vi "Periodic Tasks.vi"(8 "error in":errorcluster) -> ()   [LabVIEW 2013]
doc: "This VI runs in parallel to other tasks. It can contain as many user-defined periodic loops as you need. These can carry out PID or other sorts of timed response."
uses:
  <vilib>/Rock Robotics/SystemInterfaces/Utilities/FPGA_UtilitiesLED Source.ctl
  <vilib>/Rock Robotics/SystemInterfaces/Utilities/FPGA_UtilitiesLED State.ctl
  <vilib>/Rock Robotics/WPI/DriverStation/DriverStationLCD/WPI_DriverStationLCDLCDLine.ctl
  Robot Global Data.vi
panel:
  in  "DesiredPos 2":dbl
  in  "Deadband 2":dbl=0.2
  in  "P Gain 2":dbl=1.0
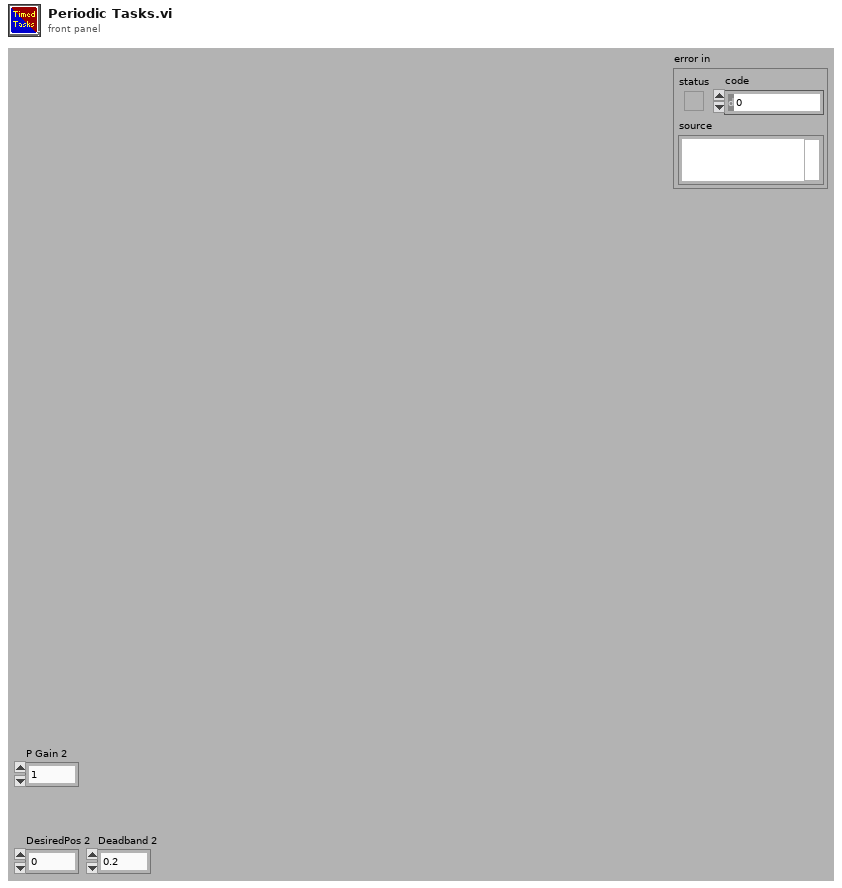
[diagram p1: front panel]
types:
  T1 = typedef "WPI_AnalogChannelDevRef.ctl" = cluster{"DevStatus":errorcluster, "Analog Module":T2, "Analog Channel":T3}
  T2 = typedef "FPGA_TypedefAnalogModule.ctl" = enum16{"Analog Module 1", "Analog Module 2"}
  T3 = typedef "FPGA_AIChannel.ctl" = enum8{"AI 1", "AI 2", "AI 3", "AI 4", "AI 5", "AI 6", "AI 7", "AI 8", "Invalid"}
  T4 = typedef "WPI_DigitalInputDevRef.ctl" = cluster{"DevStatus":errorcluster, "DIO Channel":T5, "Digital Module":T6}
  T5 = typedef "FPGA_DIOChannel.ctl" = enum8{"DIO 1", "DIO 2", "DIO 3", "DIO 4", "DIO 5", "DIO 6", "DIO 7", "DIO 8", "DIO 9", "DIO 10", "DIO 11", "DIO 12", "DIO 13", "DIO 14", "Invalid"}
  T6 = typedef "FPGA_TypedefDigitalModule.ctl" = enum16{"Digital Module 1", "Digital Module 2"}
  T7 = typedef "WPI_EncoderDevRef.ctl" = cluster{"DevStatus":errorcluster, "EncoderIndex":T8, "CounterIndex":T9, "DistancePerCount":dbl, "Decoding Type":T10}
  T8 = typedef "FPGA_EncoderIdx.ctl" = enum8{"Enc 0", "Enc 1", "Enc 2", "Enc 3", "Invalid"}
  T9 = typedef "FPGA_CounterCtrSystemIndex.ctl" = enum8{"Ctr 0", "Ctr 1", "Ctr 2", "Ctr 3", "Ctr 4", "Ctr 5", "Ctr 6", "Ctr 7", "Invalid"}
  T10 = typedef "WPI_EncoderType.ctl" = enum16{"1x", "2x", "4x"}
  T11 = cluster{"Winch Desired Location":dbl, "Winch Desired Location 2":dbl, "Winch Desired Location 3":dbl}
  T12 = typedef "FPGA_UtilitiesLED State.ctl" = enum16{"Off", "On", "Toggle"}
  T13 = typedef "FPGA_UtilitiesLED Source.ctl" = enum16{"User LED", "FPGA LED"}
  T14 = typedef "WPI_DriverStationLCDLCDLine.ctl" = enum16{"Main - Line 1", "User - Line 2", "User - Line 3", "User - Line 4", "User - Line 5", "User - Line 6"}
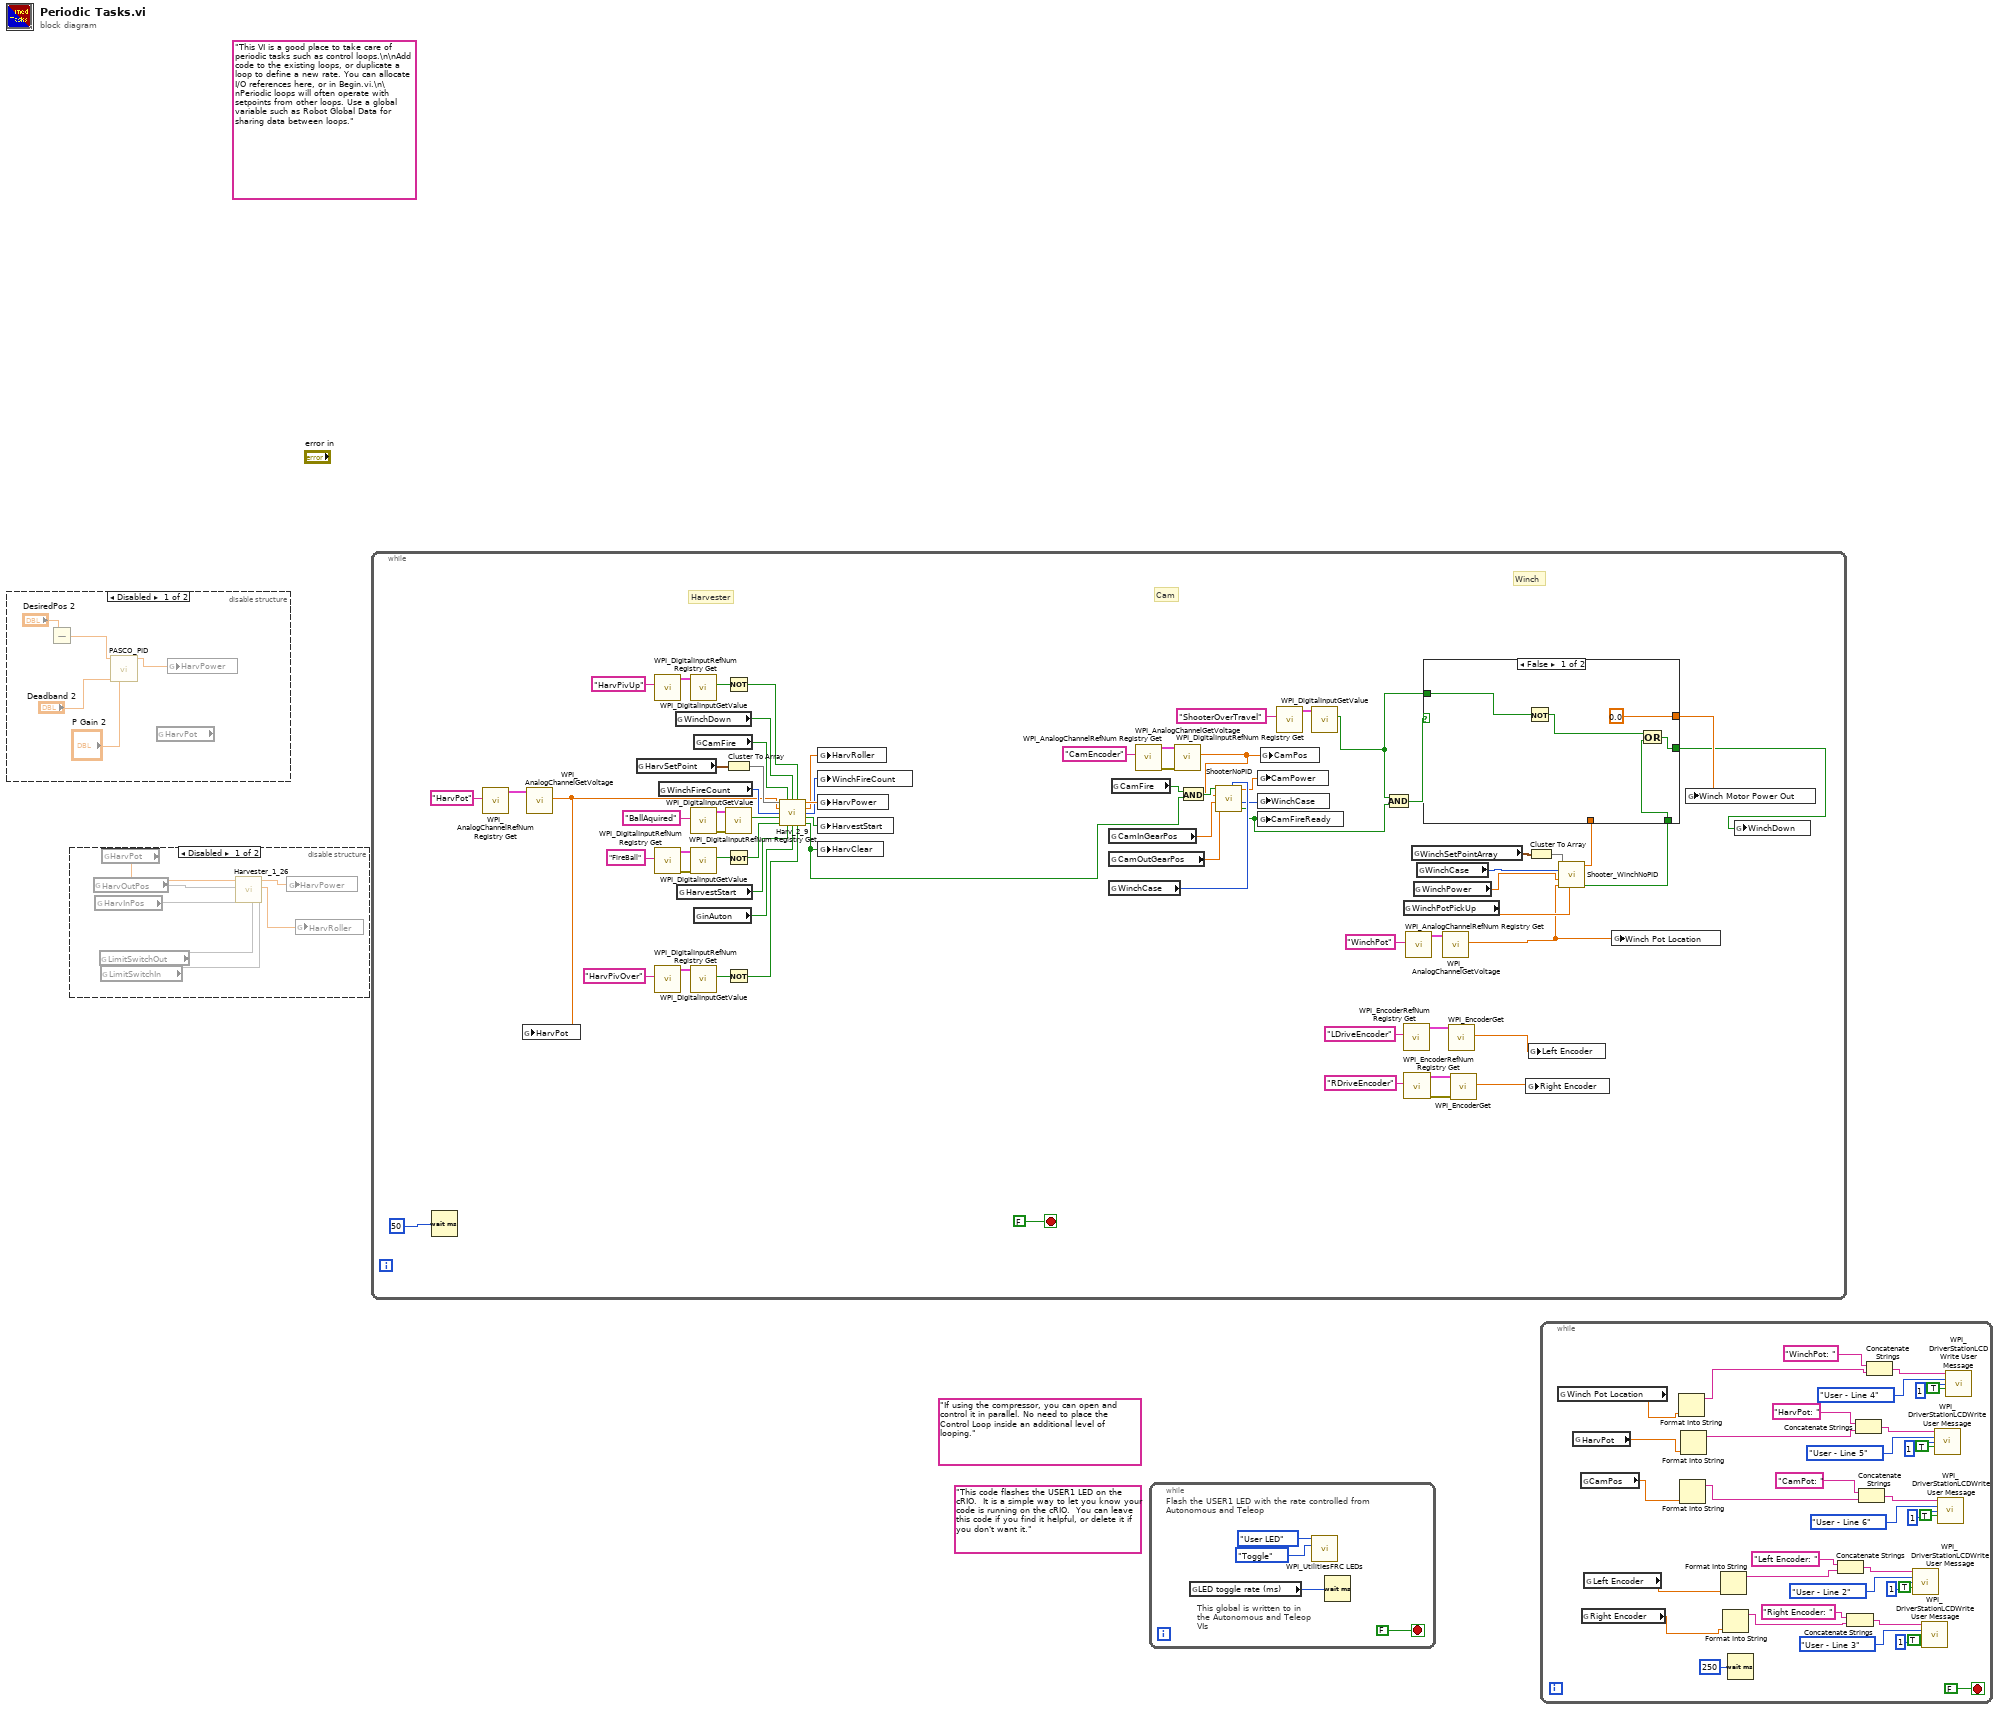
[diagram p0: block diagram]
diagram:
  (unwired) "If using the compressor, you can open and control it in parallel. No need to place the Control Loop inside an additional level of looping."
  (unwired) "This code flashes the USER1 LED on the cRIO.  It is a simple way to let you know your code is running on the cRIO.  You can leave this code if you find it helpful, or delete it if you don't want it."
  (unwired) "This VI is a good place to take care of periodic tasks such as control loops.\n\nAdd code to the existing loops, or duplicate a loop to define a new rate. You can allocate I/O references here, or in Begin.vi.\n\nPeriodic loops will often operate with setpoints from other loops. Use a global variable such as Robot Global Data for sharing data between loops."
  n1 = disable-structure shown="Disabled" {
    frame Disabled {
      n2 = Subtract(x="DesiredPos 2") -> (y=w6:dbl, x-y=w1:dbl)
      n3 = call "PASCO_PID.vi"("Delta"=w1, "Deadband"="Deadband 2", "P Gain"="P Gain 2") -> ("Output"=w3:dbl)  [unwired: 11 in, 1 out]
      n4 = global read "Robot Global Data.vi" "HarvPot"() -> (w5:dbl)
      n5 = global write "Robot Global Data.vi" "HarvPower"(w3) -> ()
    }
    frame Enabled {
    }
  }
  n6 = disable-structure shown="Disabled" {
    frame Disabled {
      n7 = global read "Robot Global Data.vi" "HarvOutPos"() -> (w13)
      n8 = global read "Robot Global Data.vi" "HarvInPos"() -> (w12)
      n9 = global read "Robot Global Data.vi" "LimitSwitchOut"() -> (w11)
      n10 = global read "Robot Global Data.vi" "LimitSwitchIn"() -> (w10)
      n11 = global read "Robot Global Data.vi" "HarvPot"() -> (w14:dbl)
      n12 = call "Harvester_1_26.vi"("LimitSwitchIn"=w10, "LimitSwitchOut"=w11, "HarvInPos"=w12, "HarvOutPos"=w13, "HarvPot"=w14) -> ("HarvRoller"=w9:dbl, "HarvPower"=w8:dbl)  [unwired: 5 in]
      n13 = global write "Robot Global Data.vi" "HarvPower"(w8) -> ()
      n14 = global write "Robot Global Data.vi" "HarvRoller"(w9) -> ()
    }
    frame Enabled {
    }
  }
  n15 = while {
    stop <- FALSE stop-if-true
    # "Winch"
    # "Cam"
    # "Harvester"
    n16 = Wait (ms)(milliseconds to wait=u32 50) -> ()  [unwired: 1 out]
    n17 = call <vilib>:"WPI_AnalogChannelRefNum Registry Get.vi"("refnum name"="HarvPot") -> ("AIDeviceRef"=w82:T1)  [unwired: 9 in, 1 out]
    n18 = call <vilib>:"WPI_AnalogChannelGetVoltage.vi"("AIDeviceRef"=w82) -> ("Voltage"=w21:dbl)  [unwired: 8 in, 2 out]
    n19 = global write "Robot Global Data.vi" "HarvPot"(w21) -> ()
    n20 = global read "Robot Global Data.vi" "HarvSetPoint"() -> (w49:cluster{"Out":dbl, "In":dbl, "Clear":dbl})
    n21 = call <vilib>:"WPI_DigitalInputRefNum Registry Get.vi"("refnum name"="HarvPivUp") -> ("DigitalInputDevRef"=w66:T4)  [unwired: 9 in, 1 out]
    n22 = call <vilib>:"WPI_DigitalInputRefNum Registry Get.vi"("refnum name"="FireBall") -> ("error out"=w55:errorcluster, "DigitalInputDevRef"=w56:T4)  [unwired: 9 in]
    n23 = call <vilib>:"WPI_DigitalInputRefNum Registry Get.vi"("refnum name"="HarvPivOver") -> ("DigitalInputDevRef"=w74:T4)  [unwired: 9 in, 1 out]
    n24 = global read "Robot Global Data.vi" "WinchFireCount"() -> (w24:i32)
    n25 = global read "Robot Global Data.vi" "WinchDown"() -> (w42:bool)
    n26 = global read "Robot Global Data.vi" "HarvestStart"() -> (w53:bool)
    n27 = call <vilib>:"WPI_DigitalInputGetValue.vi"("DigitalInputDevRef"=w66) -> ("Value"=w45:bool)  [unwired: 8 in, 2 out]
    n28 = call <vilib>:"WPI_DigitalInputRefNum Registry Get.vi"("refnum name"="BallAquired") -> ("error out"=w62:errorcluster, "DigitalInputDevRef"=w61:T4)  [unwired: 9 in]
    n29 = call <vilib>:"WPI_DigitalInputGetValue.vi"("error in (no error)"=w55, "DigitalInputDevRef"=w56) -> ("Value"=w52:bool)  [unwired: 7 in, 2 out]
    n30 = call <vilib>:"WPI_DigitalInputGetValue.vi"("DigitalInputDevRef"=w74) -> ("Value"=w47:bool)  [unwired: 8 in, 2 out]
    n31 = global read "Robot Global Data.vi" "CamFire"() -> (w54:bool)
    n32 = global read "Robot Global Data.vi" "inAuton"() -> (w26:bool)
    n33 = Not(x=w45) -> (.not. x?=w44:bool)
    n34 = Cluster To Array(cluster=w49) -> (array=w48:dbl[])
    n35 = call <vilib>:"WPI_DigitalInputGetValue.vi"("error in (no error)"=w62, "DigitalInputDevRef"=w61) -> ("Value"=w51:bool)  [unwired: 7 in, 2 out]
    n36 = Not(x=w52) -> (.not. x?=w50:bool)
    n37 = Not(x=w47) -> (.not. x?=w46:bool)
    n38 = call "Harv_2_9.vi"("HarvSetpoints"=w48, "Fire"=w54, "WinchDown"=w42, "HarvPivUP"=w44, "HarvPot"=w21, "Count"=w24, "BallAcquired"=w51, "FireBallSen"=w50, "Harvest"=w53, "inAuton?"=w26, "HarvPivPickupLim"=w46) -> ("HarvPower"=w59:dbl, "HarvRoller"=w58:dbl, "CountOut"=w23:i32, "HarvStart"=w43:bool, "HarvCleared"=w20:bool)
    n39 = global write "Robot Global Data.vi" "HarvRoller"(w58) -> ()
    n40 = global write "Robot Global Data.vi" "WinchFireCount"(w23) -> ()
    n41 = global write "Robot Global Data.vi" "HarvPower"(w59) -> ()
    n42 = global write "Robot Global Data.vi" "HarvestStart"(w43) -> ()
    n43 = global write "Robot Global Data.vi" "HarvClear"(w20) -> ()
    n44 = global read "Robot Global Data.vi" "CamInGearPos"() -> (w31:dbl)
    n45 = global read "Robot Global Data.vi" "CamOutGearPos"() -> (w30:dbl)
    n46 = global read "Robot Global Data.vi" "WinchCase"() -> (w32:i32)
    n47 = global read "Robot Global Data.vi" "CamFire"() -> (w68:bool)
    n48 = call <vilib>:"WPI_AnalogChannelRefNum Registry Get.vi"("refnum name"="CamEncoder") -> ("error out"=w70:errorcluster, "AIDeviceRef"=w69:T1)  [unwired: 9 in]
    n49 = call <vilib>:"WPI_AnalogChannelGetVoltage.vi"("error in (no error)"=w70, "AIDeviceRef"=w69) -> ("Voltage"=w19:dbl)  [unwired: 7 in, 2 out]
    n50 = And(x=w68, y=w20) -> (x .and. y?=w33:bool)
    n51 = call "ShooterNoPID.vi"("WinchCaseIn"=w32, "InGearPosLow"=w30, "InGearPosHigh"=w31, "Pot"=w19, "Fire"=w33) -> ("There?"=w27:bool, "WinchCase"=w28:i32, "Power"=w29:dbl)  [unwired: 4 in]
    n52 = global write "Robot Global Data.vi" "CamPower"(w29) -> ()
    n53 = global write "Robot Global Data.vi" "WinchCase"(w28) -> ()
    n54 = global write "Robot Global Data.vi" "CamFireReady"(w27) -> ()
    n55 = global write "Robot Global Data.vi" "CamPos"(w19) -> ()
    n56 = call <vilib>:"WPI_DigitalInputRefNum Registry Get.vi"("refnum name"="ShooterOverTravel") -> ("DigitalInputDevRef"=w65:T4)  [unwired: 9 in, 1 out]
    n57 = call <vilib>:"WPI_DigitalInputGetValue.vi"("DigitalInputDevRef"=w65) -> ("Value"=w41:bool)  [unwired: 8 in, 2 out]
    n58 = And(x=w41, y=w27) -> (x .and. y?=w63:bool)
    n59 = global read "Robot Global Data.vi" "WinchPotPickUp"() -> (w25:dbl)
    n60 = call <vilib>:"WPI_EncoderRefNum Registry Get.vi"("refnum name"="LDriveEncoder") -> ("EncoderDevRef"=w76:T7)  [unwired: 9 in, 1 out]
    n61 = call <vilib>:"WPI_EncoderRefNum Registry Get.vi"("refnum name"="RDriveEncoder") -> ("error out"=w18:errorcluster, "EncoderDevRef"=w17:T7)  [unwired: 9 in]
    n62 = call <vilib>:"WPI_AnalogChannelRefNum Registry Get.vi"("refnum name"="WinchPot") -> ("AIDeviceRef"=w78:T1)  [unwired: 9 in, 1 out]
    n63 = global read "Robot Global Data.vi" "WinchSetPointArray"() -> (w38:T11)
    n64 = global read "Robot Global Data.vi" "WinchPower"() -> (w40:dbl)
    n65 = global read "Robot Global Data.vi" "WinchCase"() -> (w37:i32)
    n66 = call <vilib>:"WPI_AnalogChannelGetVoltage.vi"("AIDeviceRef"=w78) -> ("Voltage"=w22:dbl)  [unwired: 8 in, 2 out]
    n67 = call <vilib>:"WPI_EncoderGet.vi"("EncoderDevRef"=w76) -> ("Distance"=w16:dbl)  [unwired: 5 in, 5 out]
    n68 = call <vilib>:"WPI_EncoderGet.vi"("error in (no error)"=w18, "EncoderDevRef"=w17) -> ("Distance"=w15:dbl)  [unwired: 4 in, 5 out]
    n69 = global write "Robot Global Data.vi" "Right Encoder"(w15) -> ()
    n70 = Cluster To Array(cluster=w38) -> (array=w39:dbl[])
    n71 = global write "Robot Global Data.vi" "Left Encoder"(w16) -> ()
    n72 = call "Shooter_WinchNoPID.vi"("PickStartPos"=w25, "Winch Pot Location"=w22, "WinchPower"=w40, "selectedCase"=w37, "SetPointArray"=w39) -> ("isThere?"=w35:bool, "Winch Motor Power Out"=w34:dbl)  [unwired: 5 in]
    n73 = case shown="False" w63 {
      tunnel: [0.0 ("Winch Motor Power Out") w89] -> w72
      tunnel: [w87 w90] -> w36
      tunnel: w41 -> [w86 _]
      tunnel: w35 -> [w84 w90]
      tunnel: w34 -> [_ w89]
      frame False {
        n74 = Not(x=w86) -> (.not. x?=w85:bool)
        n75 = Or(x=w85, y=w84) -> (x .or. y?=w87:bool)
      }
      frame True {
      }
    }
    n76 = global write "Robot Global Data.vi" "Winch Pot Location"(w22) -> ()
    n77 = global write "Robot Global Data.vi" "Winch Motor Power Out"(w72) -> ()
    n78 = global write "Robot Global Data.vi" "WinchDown"(w36) -> ()
  }
  n79 = while {
    stop <- FALSE stop-if-true
    # "This global is written to in the Autonomous and Teleop VIs"
    # "Flash the USER1 LED with the rate controlled from Autonomous and Teleop"
    n80 = global read "Robot Global Data.vi" "LED toggle rate (ms)"() -> (w91:u32)
    n81 = call <vilib>:"WPI_UtilitiesFRC LEDs.vi"("State"=FPGA_UtilitiesLED_State."Toggle", "LED Type"=FPGA_UtilitiesLED_Source."User LED") -> ()  [unwired: 1 in, 9 out]
    n82 = Wait (ms)(milliseconds to wait=w91) -> ()  [unwired: 1 out]
  }
  n83 = while {
    stop <- FALSE stop-if-true
    n84 = global read "Robot Global Data.vi" "Winch Pot Location"() -> (w100:dbl)
    n85 = global read "Robot Global Data.vi" "HarvPot"() -> (w99:dbl)
    n86 = global read "Robot Global Data.vi" "CamPos"() -> (w101:dbl)
    n87 = global read "Robot Global Data.vi" "Right Encoder"() -> (w97:dbl)
    n88 = global read "Robot Global Data.vi" "Left Encoder"() -> (w98:dbl)
    n89 = Format Into String(w100) -> (resulting string=w117:string)  [unwired: 3 in, 1 out]
    n90 = Format Into String(w101) -> (resulting string=w102:string)  [unwired: 3 in, 1 out]
    n91 = Format Into String(w99) -> (resulting string=w111:string)  [unwired: 3 in, 1 out]
    n92 = Format Into String(w98) -> (resulting string=w109:string)  [unwired: 3 in, 1 out]
    n93 = Format Into String(w97) -> (resulting string=w108:string)  [unwired: 3 in, 1 out]
    n94 = Wait (ms)(milliseconds to wait=u32 250) -> ()  [unwired: 1 out]
    n95 = Concatenate Strings("Left Encoder: ", w109) -> (w127:string)
    n96 = Concatenate Strings("Right Encoder: ", w108) -> (w126:string)
    n97 = Concatenate Strings("HarvPot: ", w111) -> (w112:string)
    n98 = Concatenate Strings("CamPot: ", w102) -> (w107:string)
    n99 = Concatenate Strings("WinchPot: ", w117) -> (w122:string)
    n100 = call <vilib>:"WPI_DriverStationLCDWrite User Message.vi"("line text"=w127, "line"=WPI_DriverStationLCDLCDLine."User - Line 2", "starting column"=i8 1, "clear line before write (T)"=TRUE) -> ()  [unwired: 1 in, 11 out]
    n101 = call <vilib>:"WPI_DriverStationLCDWrite User Message.vi"("line text"=w126, "line"=WPI_DriverStationLCDLCDLine."User - Line 3", "starting column"=i8 1, "clear line before write (T)"=TRUE) -> ()  [unwired: 1 in, 11 out]
    n102 = call <vilib>:"WPI_DriverStationLCDWrite User Message.vi"("line text"=w112, "line"=WPI_DriverStationLCDLCDLine."User - Line 5", "starting column"=i8 1, "clear line before write (T)"=TRUE) -> ()  [unwired: 1 in, 11 out]
    n103 = call <vilib>:"WPI_DriverStationLCDWrite User Message.vi"("line text"=w107, "line"=WPI_DriverStationLCDLCDLine."User - Line 6", "starting column"=i8 1, "clear line before write (T)"=TRUE) -> ()  [unwired: 1 in, 11 out]
    n104 = call <vilib>:"WPI_DriverStationLCDWrite User Message.vi"("line text"=w122, "line"=WPI_DriverStationLCDLCDLine."User - Line 4", "starting column"=i8 1, "clear line before write (T)"=TRUE) -> ()  [unwired: 1 in, 11 out]
  }
